vi "Test MQTT-4.7.1-3.vi"(8 "error in (no error)":errorcluster) -> (0 "error out":errorcluster)   [LabVIEW 2013]
uses:
  <vilib>/addons/_JKI Toolkits/Caraya/classes/Test/Test.lvclass
  <vilib>/addons/_JKI Toolkits/Caraya/classes/Assert/Assert.lvclass
  <vilib>/LabVIEW Open Source Project/MQTT Connection/MQTT_Base/TopicFilter/TopicFilter.lvclass
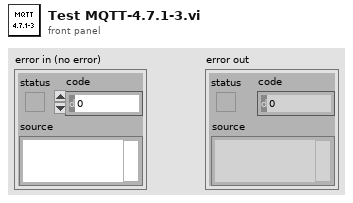
[diagram p1: front panel]
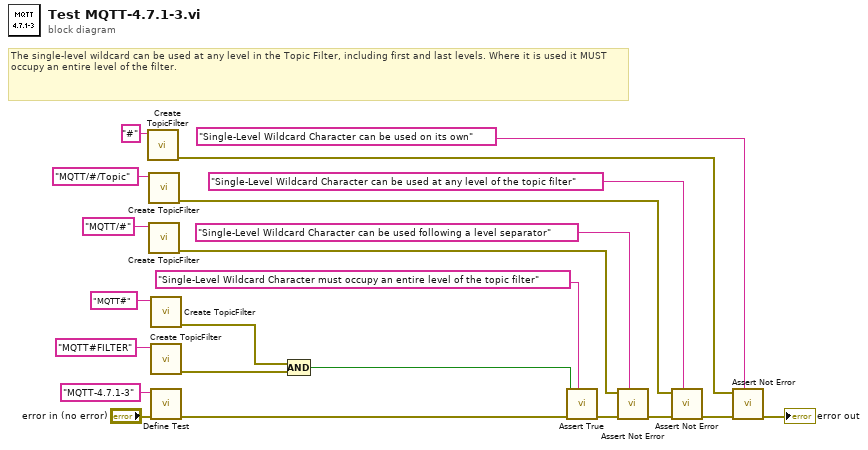
[diagram p0: block diagram]
diagram:
  # "The single-level wildcard can be used at any level in the Topic Filter, including first and last levels. Where it is used it MUST occupy an entire level of the filter."
  n1 = call <vilib>:"Create TopicFilter.vi"("Topic Filter"="#" ("Topic Name")) -> ("error out"=w10:errorcluster)  [unwired: 9 in, 1 out]
  n2 = call <vilib>:"Create TopicFilter.vi"("Topic Filter"="MQTT/#/Topic" ("Topic Name")) -> ("error out"=w5:errorcluster)  [unwired: 9 in, 1 out]
  n3 = call <vilib>:"Create TopicFilter.vi"("Topic Filter"="MQTT/#" ("Topic Name")) -> ("error out"=w6:errorcluster)  [unwired: 9 in, 1 out]
  n4 = call <vilib>:"Create TopicFilter.vi"("Topic Filter"="MQTT#" ("Topic Name")) -> ("error out"=w2:errorcluster)  [unwired: 9 in, 1 out]
  n5 = call <vilib>:"Create TopicFilter.vi"("Topic Filter"="MQTT#FILTER" ("Topic Name")) -> ("error out"=w3:errorcluster)  [unwired: 9 in, 1 out]
  n6 = call <vilib>:"Define Test.vi"("error in (no error)"="error in (no error)", "Label (VI Title)"="MQTT-4.7.1-3") -> ("error out"=w19:errorcluster)  [unwired: 9 in]
  n7 = Compound Arithmetic op=AND(w2, w3) -> (w1:bool)
  n8 = call <vilib>:"Assert True.vi"("Label"="Single-Level Wildcard Character must occupy an entire level of the topic filter", "error in (no error)"=w19, "True?"=w1) -> ("error out"=w15:errorcluster)  [unwired: 8 in]
  n9 = call <vilib>:"Assert Not Error.vi"("Label"="Single-Level Wildcard Character can be used following a level separator", "error in (no error)"=w15, "Not Error?"=w6) -> ("error out"=w14:errorcluster)  [unwired: 8 in]
  n10 = call <vilib>:"Assert Not Error.vi"("Label"="Single-Level Wildcard Character can be used at any level of the topic filter", "error in (no error)"=w14, "Not Error?"=w5) -> ("error out"=w17:errorcluster)  [unwired: 8 in]
  n11 = call <vilib>:"Assert Not Error.vi"("Label"="Single-Level Wildcard Character can be used on its own", "error in (no error)"=w17, "Not Error?"=w10) -> ("error out"=→"error out":errorcluster)  [unwired: 8 in]
